vi "chart add series lv.vi"(8 "error in (no error)":errorcluster, 9 "values":string, 10 "categories":string, 11 "chart":u32) -> (0 "error out":errorcluster, 3 "function return":u32)   [LabVIEW 2015, in "xlsxwriter.lvlib"]
doc: "lxw_chart_series chart_add_series_lv(lxw_chart chart, const char *categories, const char *values);"
uses:
  xlsxwriter.lvlib
  xlsxwriter.dll
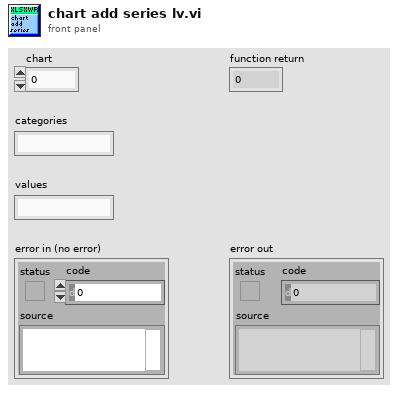
[diagram p1: front panel]
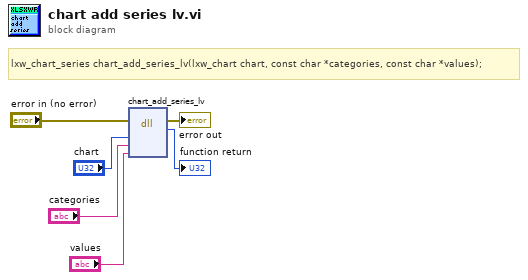
[diagram p0: block diagram]
diagram:
  # "lxw_chart_series chart_add_series_lv(lxw_chart chart, const char *categories, const char *values);"
  n1 = dll-call lib="C:/Users/WDAGUtilityAccount/Desktop/lv_vis_added_cell/xlsxwriter.*" fn="chart_add_series_lv"(error in="error in (no error)", "chart"="chart", "categories"="categories", "values"="values") -> (error out=→"error out":errorcluster, →"function return":u32)  [unwired: 5 in, 1 out]
